vi "KE6221 -- PDelta Mode Set Num Cycles.vi"(0 "Resource In":refnum<visa-resource-name>, 1 "Check For SCPI Errors? (T)":bool=TRUE, 5 "Num Cycles Mode":T1, 7 "Finite Count":T2=1 min=1 max=65536, 11 "error in (no error)":errorcluster) -> (4 "Resource Out (dupl)":refnum<visa-resource-name>, 15 "error out":errorcluster)   [LabVIEW 2019, in "Keithley 622x.lvlib"]
uses:
  Keithley 622x.lvlib
  Typedefs/KE622x -- Delta PDelta Mode Num Cycles.ctl
  Typedefs/KE622x -- Delta PDelta Mode Num Cycles Mode.ctl
panel:
  # "*** NOTE:  \"Finite Count\" is ignored\nif \"Num Cycles Mode\" is 'Infinite'."
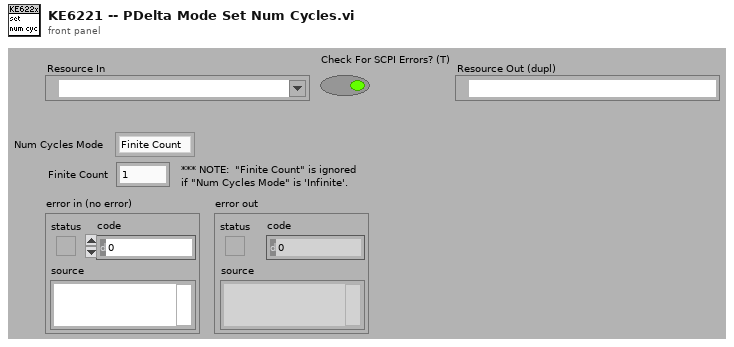
[diagram p1: front panel]
types:
  T1 = typedef "Keithley 622x.lvlib/KE622x -- Delta PDelta Mode Num Cycles Mode.ctl" = enum16{"Finite Count", "Infinite"}
  T2 = typedef "Keithley 622x.lvlib/KE622x -- Delta PDelta Mode Num Cycles.ctl" = u32
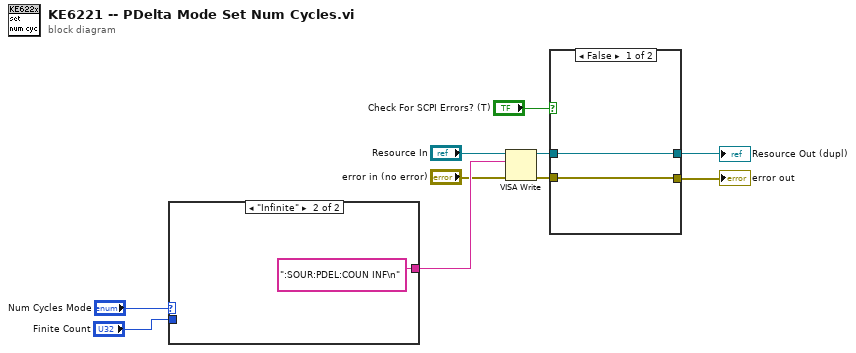
[diagram p0: block diagram]
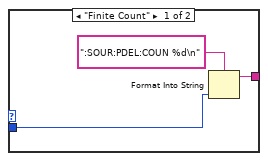
[diagram p2: hidden frame]
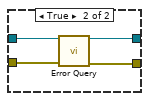
[diagram p3: hidden frame]
diagram:
  n1 = case shown="\"Infinite\"" "Num Cycles Mode" {
    tunnel: [w12 ":SOUR:PDEL:COUN INF\n"] -> w9
    tunnel: "Finite Count" -> [w11 _]
    frame "Finite Count" {
      n2 = Format Into String(format string=":SOUR:PDEL:COUN %d\n", w11) -> (resulting string=w12:string)  [unwired: 2 in, 1 out]
    }
    frame "Infinite" {
    }
  }
  n3 = VISA Write(VISA resource name="Resource In", write buffer=w9, error in (no error)="error in (no error)") -> (VISA resource name out=w6:refnum<visa-resource-name>, error out=w5:errorcluster)  [unwired: 1 out]
  n4 = case shown="False" "Check For SCPI Errors? (T)" {
    tunnel: w6 -> [w16 w20]
    tunnel: w5 -> [w15 w19]
    tunnel: [w15 w18] -> w1
    tunnel: [w16 w17] -> w2
    frame False {
    }
    frame True {
      n5 = call "Error Query.vi"("VISA Resource In"=w20, "error in (no error)"=w19) -> ("VISA Resource Out (dupl)"=w17:refnum<visa-resource-name>, "error out"=w18:errorcluster)  [unwired: 10 in, 2 out]
    }
  }
  "Resource Out (dupl)" <- w2
  "error out" <- w1
